vi "Clear Snapshot.vi"(8 "error in":errorcluster, 11 "Electronic Load in":refnum<class "Electronic Load.lvclass">) -> (0 "error out":errorcluster, 3 "Electronic Load out":refnum<class "Electronic Load.lvclass">)   [LabVIEW 2019, in "Electronic Load.lvlib" / "Electronic Load.lvclass"]
uses:
  Library/Electronic Load.lvclass
  C:/Users/Public/Documents/Development/builds/Instruments/Instruments.lvlibp/Library/Instruments.lvclass
  builds/Instruments/Instruments.lvlibp/Accessors/Read Snapshot Refnum.vi
  builds/Instruments/Instruments.lvlibp/Accessors/Write Snapshot Refnum.vi
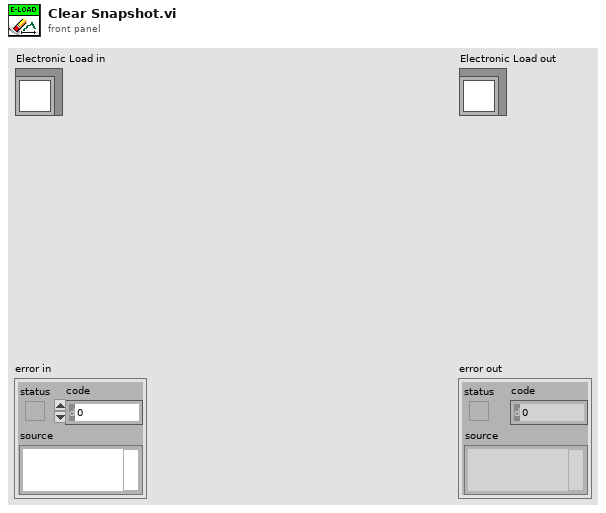
[diagram p1: front panel]
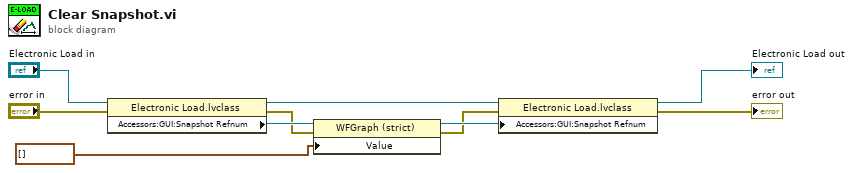
[diagram p0: block diagram]
diagram:
  n1 = property class="Electronic Load.lvclass"(reference="Electronic Load in", error in="error in") -> (reference out=w8:refnum<class "Electronic Load.lvclass">, error out=w4:errorcluster, "Accessors:GUI:Snapshot Refnum"=w7:refnum<vi>)
  n2 = property class="WFGraph (strict)"(reference=w7, error in=w4, "Value"=waveform(dbl)[] []) -> (reference out=w6:refnum<vi>, error out=w3:errorcluster)
  n3 = property class="Electronic Load.lvclass"(reference=w8, error in=w3, "Accessors:GUI:Snapshot Refnum"=w6) -> (reference out=→"Electronic Load out":refnum<class "Electronic Load.lvclass">, error out=→"error out":errorcluster)
